vi "Window-About.vi"() -> ()   [LabVIEW 2013]
doc: "Use this template to create a dialog box with event handling."
uses:
  Typedefs/Which path.ctl
  <vilib>/Utility/miscctls.llb/LVPointTypeDef.ctl
  Program Files (x86)/National Instruments/LabVIEW 2013/user.lib/My Palettes.lib/Timestamp-Date-Time/Typedefs/SN Components Enum.ctl
  Global Variables/gl_UI Ctrl Refs.vi
  Global Variables/General Globals.vi
panel:
  out "Development years":string
  out "Revision":string
  in  "Website":bool
  # "2-Photon Microscopy Software"
  # "The Silver Lab"
  # "University College London"
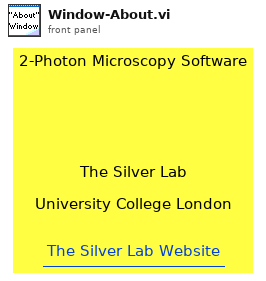
[diagram p1: front panel]
types:
  T1 = typedef "Which path.ctl" = enum16{"Configuration Files", "Calibration Files", "Images", "Setup.ini", "Loaded User profile.ini", "User's-Previous session.ini", "New user profile.ini", "Selected User profile.ini", "User profiles folder", "Power meter scaling.txt", "FOV Cal.ini"}
  T2 = typedef "SN Components Enum.ctl" = enum16{"Constant String", "Incrementing number", "Space", "Day of the week (D)", "Day of the week (DD)", "Day of the month (D)", "Day of the month (DD)", "W", "WW", "MM", "YY", "YYYY"}
  T3 = typedef "LVPointTypeDef.ctl" = cluster{"Horizontal":i16, "Vertical":i16}
  T4 = typedef "UI ctrl refs cluster.ctl" = cluster{"Top level VI path":path, "Top level VI ref":refnum<vi>, "User menu ref":refnum<k9>, "Sub Panel control":refnum<vi>, "Imaging Param Tab":refnum<vi>, "Occurrence-Start drivers":refnum<k4>, "Occurrence-Speed logging initialised":refnum<k4>, "Occurrence-XYZ stage initialised":refnum<k4>, "Exit button":refnum<vi>, "Status ind":refnum<vi>, "Return to Origin":refnum<vi>, "Speed Logging":refnum<vi>, "Time Lapse":refnum<vi>, "Live Imaging":refnum<vi>, "AOL Z Stack":refnum<vi>, "Motor Z Stack":refnum<vi>, "Funct Acq button":refnum<vi>, "Hard Shutter":refnum<vi>, "Virtual Shutter":refnum<vi>, "Laser Power":refnum<vi>, "AOL Mode":refnum<vi>, "Frame Size":refnum<vi>, "Field of View":refnum<vi>, "Dwell Time":refnum<vi>, "Zoom":refnum<vi>, "AOL Z":refnum<vi>, "Objective":refnum<vi>, "Axis":refnum<vi>, "Paths & Names":refnum<vi>, "Experiment folder path (ind.)":refnum<vi>, "Last State (Ind.)":refnum<vi>, "Laser wavelength ind (nm)":refnum<vi>, "Averages":refnum<vi>, "Angle (degrees)":refnum<vi>, "X centre":refnum<vi>, "Y centre":refnum<vi>, "Plane Mode":refnum<vi>, "# Planes":refnum<vi>, "Z Start":refnum<vi>, "Z Stop":refnum<vi>, "Z Step":refnum<vi>, "PMT 1":refnum<vi>, "PMT 2":refnum<vi>, "Stage XYZ Position":refnum<vi>, "Pockels@Z Start":refnum<vi>, "Pockels@Z Stop":refnum<vi>, "Obtain Z Start":refnum<vi>, "Obtain Z Stop":refnum<vi>, "Live stim.trig.period":refnum<vi>, "Live stim.trig.enable":refnum<vi>, "Funct. Acq. Pockels Modulation":refnum<vi>, "Enable Video Recording":refnum<vi>, "Video Record-Live Imaging":refnum<vi>, "Video Record-Funct acq":refnum<vi>, "AOL Z-stack Chirps Ready (ind)":refnum<vi>, "Center freq ind (nm)":refnum<vi>, "Logging queue (ind)":refnum<vi>, "Back aperture power (ind.)":refnum<vi>, "Power after objective (ind.)":refnum<vi>, "Switch user":refnum<vi>}
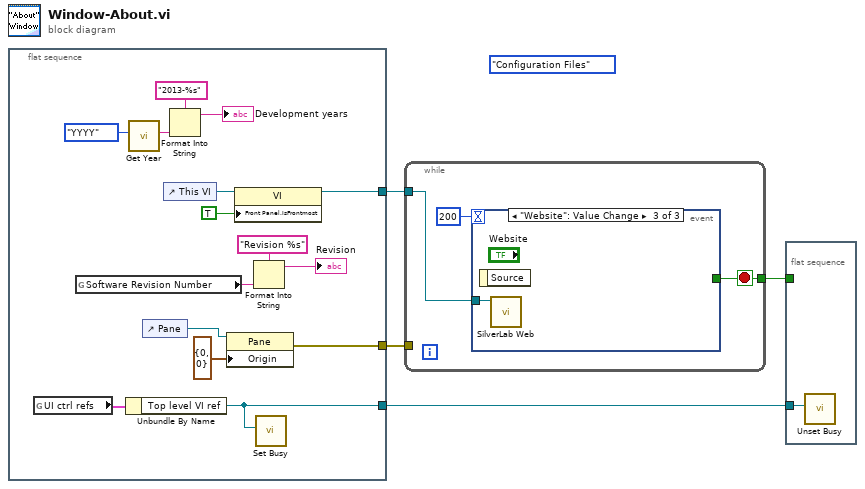
[diagram p0: block diagram]
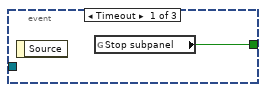
[diagram p2: hidden frame]
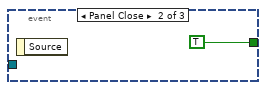
[diagram p3: hidden frame]
diagram:
  (unwired) Which_path."Configuration Files" ("Which file or folder?")
  n1 = flat-sequence {
    tunnel: [w17] -> w4
    tunnel: [w15] -> w3
    tunnel: [w12] -> w1
    frame #0 {
      n2 = global read "gl_UI Ctrl Refs.vi" "UI ctrl refs"() -> (w13:T4)
      n3 = global read "General Globals.vi" "Software Revision Number"() -> (w5:string)
      n4 = Unbundle By Name(w13) -> ("Top level VI ref"=w12:refnum<vi>)
      n5 = call "Get Year.vi"("Day format"=SN_Components_Enum."YYYY") -> ("Year"=w7:string)  [unwired: 10 in]
      n6 = control-ref of="Pane"() -> (w14:refnum<vi>)
      n7 = control-ref of="This VI"() -> (w18:refnum<vi>)
      n8 = Format Into String(format string="2013-%s", w7) -> (resulting string=→"Development years":string)  [unwired: 2 in, 1 out]
      n9 = property class="Pane"(reference=w14, "Origin"=T3 {"Horizontal"=0, "Vertical"=0}) -> (error out=w15:errorcluster)  [unwired: 1 in, 1 out]
      n10 = property on="Property Node" class="VI"(reference=w18, "Front Panel.IsFrontmost"=TRUE ("Front Panel Window:Is Frontmost")) -> (reference out=w17:refnum<vi>)  [unwired: 1 in, 1 out]
      n11 = Format Into String(format string="Revision %s", w5) -> (resulting string=→"Revision":string)  [unwired: 2 in, 1 out]
      n12 = call <vilib>:"Set Busy.vi"("VI reference (current VI)"=w12) -> ()  [unwired: 9 in, 2 out]
    }
  }
  n13 = while {
    tunnel: w3 -> [_]
    tunnel: w4 -> [w20]
    tunnel: [w21] -> w2
    stop <- w21 stop-if-true
    n14 = event shown="[2] \"Website\": Value Change" {
      selector: _ -> [_ _ _]
      dyn-events: _ -> [_ _ _]
      timeout: 200 -> [_ _ _]
      tunnel: [w23 TRUE ("Stop?") _] -> w21
      tunnel: w20 -> [_ _ w25]
      event Timeout {
        n15 = event-data() -> ()  [unwired: 1 in, 1 out]
        n16 = global read "General Globals.vi" "Stop subpanel"() -> (w23:bool)
      }
      event Panel Close {
        n17 = event-data() -> ()  [unwired: 1 in, 1 out]
      }
      event "Website": Value Change {
        n18 = event-data() -> ()  [unwired: 1 in, 1 out]
        n19 = call "SilverLab Web.vi"("Calle window's ref"=w25) -> ()  [unwired: 11 in]
      }
    }
  }
  n20 = flat-sequence {
    tunnel: w2 -> [_]
    tunnel: w1 -> [w26]
    frame #0 {
      n21 = call <vilib>:"Unset Busy.vi"("VI reference (current VI)"=w26) -> ()  [unwired: 10 in, 1 out]
    }
  }
